vi "Get 2-Exp Global Fit Guess Parameters.vi"(9 "Global Fit Data":T1={"Fit Data"=variant(cluster{"t Array":dbl[], "IRF Array":dbl[]} {"t Array"=[], "IRF Array"=[]}), "Global Fit Parameter Information"={"Original Parameter Indices"=[], "# Global Parameters"=0, "# Plot Specific Parameters"=0, "Global Parameter? Array"=[]}, "# Points in Plots"=[]}, 10 "Index Max Array":i32[](array[numeric])) -> (2 "Initial Parameters":dbl[](array[numeric])=[-1.0, 0.0, 0.5, 0.1, 0.5, 1.0])   [LabVIEW 2021, in "Fits.lvlib"]
uses:
  Fits.lvlib
  0514af7e-a1fd-4741-8e5a-4de6127bfab8.vi
  Graphs/XY Graph/XY Graph Plot Data.ctl
  Graphs/XY Graph/XY Graph Add-Ons.lvlib
  Global Fit Parameters Information.ctl
  Global Fit Data.ctl
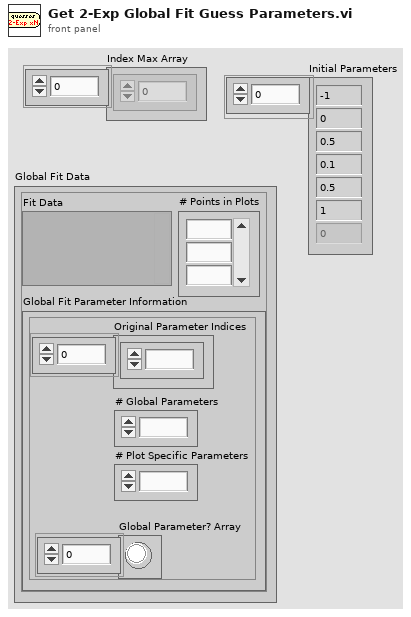
[diagram p1: front panel]
types:
  T1 = typedef "Fits.lvlib/Global Fit Data.ctl" = cluster{"Fit Data":variant, "Global Fit Parameter Information":T2, "# Points in Plots":i32[]}
  T2 = typedef "Fits.lvlib/Global Fit Parameters Information.ctl" = cluster{"Original Parameter Indices":i32[], "# Global Parameters":i32, "# Plot Specific Parameters":i32, "Global Parameter? Array":bool[]}
  T3 = typedef "XY Graph Add-Ons.lvlib/XY Graph Plot Data.ctl" = cluster{"X Array":dbl[], "Y Array":dbl[]}
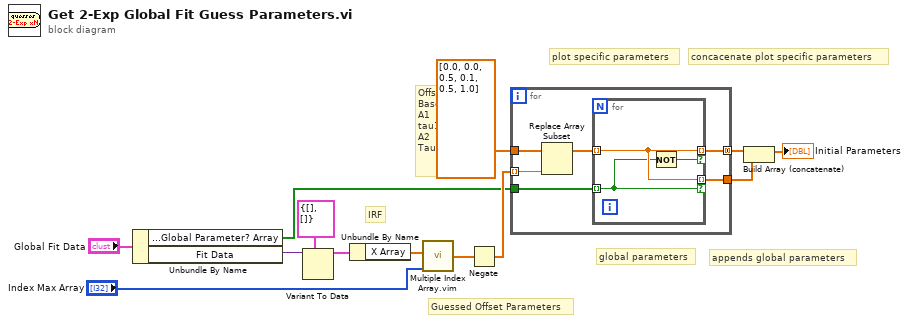
[diagram p0: block diagram]
diagram:
  # "Offset\nBaseline\nA1\ntau1\nA2\nTau2"
  # "Guessed Offset Parameters"
  # "IRF"
  # "appends global parameters"
  # "concacenate plot specific parameters"
  # "plot specific parameters"
  # "global parameters"
  n1 = Unbundle By Name("Global Fit Data") -> ("Global Fit Parameter Information.Global Parameter? Array"=w3:bool[], "Fit Data"=w12:variant)
  n2 = Variant To Data(type=T3 {"X Array"=[], "Y Array"=[]} ("Plot"), Variant=w12) -> (data=w4:T3)  [unwired: 1 in, 1 out]
  n3 = Unbundle By Name(w4) -> ("X Array"=w5:dbl[])
  n4 = call "Multiple Index Array.vim"("Index Array"="Index Max Array", "Array"=w5) -> ("Selected Element(s)"=w10:dbl[])  [unwired: 4 in]
  n5 = Negate(x=w10) -> (-x=w9:dbl[])
  n6 = for {
    tunnel: dbl[] [0.0, 0.0, 0.5, 0.1, 0.5, 1.0] ("Initial Parameters") -> [w19]
    tunnel: [w15] -> w11 mode=concatenating
    tunnel: w9 -> [w18] mode=indexing
    tunnel: w3 -> [w17]
    tunnel: [w14] -> w1
    n7 = Replace Array Subset(array=w19, new element=w18) -> (w16:dbl[])  [unwired: 1 in]
    n8 = for {
      tunnel: w17 -> [w21] mode=indexing
      tunnel: w16 -> [w22] mode=indexing
      tunnel: [w22] -> w14 mode=indexing if=w21
      tunnel: [w22] -> w15 mode=indexing if=w20
      n9 = Not(x=w21) -> (.not. x?=w20:bool)
    }
  }
  n10 = Build Array (concatenate)(w11, w1) -> (→"Initial Parameters":dbl[])
